vi "Get Tables for Testing.vi"(8 "error in (no error)":errorcluster, 11 "Update Fields Logic Simple Table in":refnum<class "Update Fields Logic Simple Table.lvclass">) -> (0 "error out":errorcluster, 1 "FK Column":string[](array[string]), 2 "FK Table":string[](array[string]), 3 "Update Fields Logic Simple Table out":refnum<class "Update Fields Logic Simple Table.lvclass">, 4 "PK Column":string[](array[string]), 5 "Field ID":string[](array[string]), 6 "PK Table":string[](array[string]), 7 "Form IDs":T1[](array[typedef]))   [LabVIEW 2020, in "Update Fields Logic Simple Table.lvlib" / "Update Fields Logic Simple Table.lvclass"]
uses:
  Update Fields Logic Simple Table.lvclass
  Form ID.ctl
  Update Fields Logic Simple Table.lvclass/Update Fields Logic Simple Table.ctl
  Form Server Interfaces.lvlib
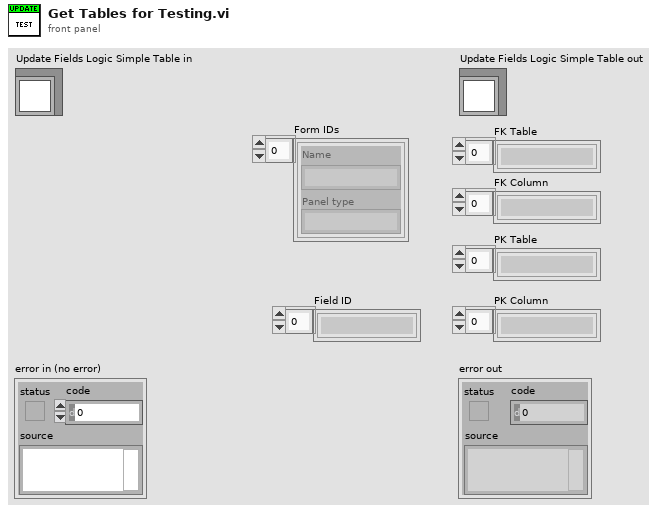
[diagram p1: front panel]
types:
  T1 = typedef "Form Server Interfaces.lvlib/Form ID.ctl" = cluster{"Name":string, "Panel type":string}
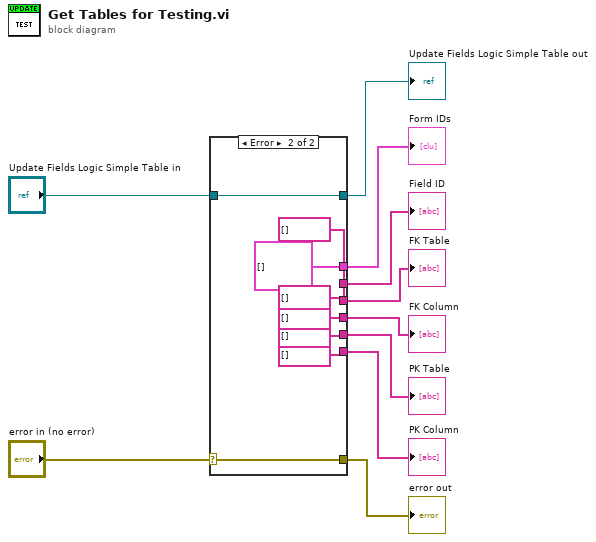
[diagram p0: block diagram]
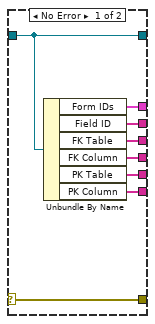
[diagram p2: hidden frame]
diagram:
  n1 = case shown="Error" "error in (no error)" {
    selector: "error in (no error)" -> [w18 w26]
    tunnel: [w18 w26] -> w9
    tunnel: [w17 w25] -> w7
    tunnel: "Update Fields Logic Simple Table in" -> [w17 w25]
    tunnel: [w16 T1[] [] ("Form IDs")] -> w6
    tunnel: [w15 string[] [] ("Field ID")] -> w5
    tunnel: [w14 string[] [] ("FK Table")] -> w4
    tunnel: [w13 string[] [] ("FK Column")] -> w3
    tunnel: [w12 string[] [] ("PK Table")] -> w2
    tunnel: [w11 string[] [] ("PK Column")] -> w1
    frame No Error {
      n2 = Unbundle By Name(w17) -> ("Form IDs"=w16:T1[], "Field ID"=w15:string[], "FK Table"=w14:string[], "FK Column"=w13:string[], "PK Table"=w12:string[], "PK Column"=w11:string[])
    }
    frame Error {
    }
  }
  "error out" <- w9
  "Update Fields Logic Simple Table out" <- w7
  "Form IDs" <- w6
  "Field ID" <- w5
  "FK Table" <- w4
  "FK Column" <- w3
  "PK Table" <- w2
  "PK Column" <- w1
